vi "get_node_attribute.vi"(7 "attribute-name":string, 8 "error in (no error)":errorcluster, 9 "default value (empty variant)":variant, 10 "node":refnum<class "Node.lvclass">, 11 "graph":refnum<class "Graph.lvclass">) -> (0 "error out":errorcluster, 1 "attribute-value":variant, 2 "attribute found":bool, 3 "graph-out":refnum<class "Graph.lvclass">)   [LabVIEW 2020, in "graph.lvlib" / "Graph.lvclass"]
uses:
  Graph.lvclass
  Node/Node.lvclass
  Node/Node.lvclass/Node.ctl
  Graph.lvclass/Graph.ctl
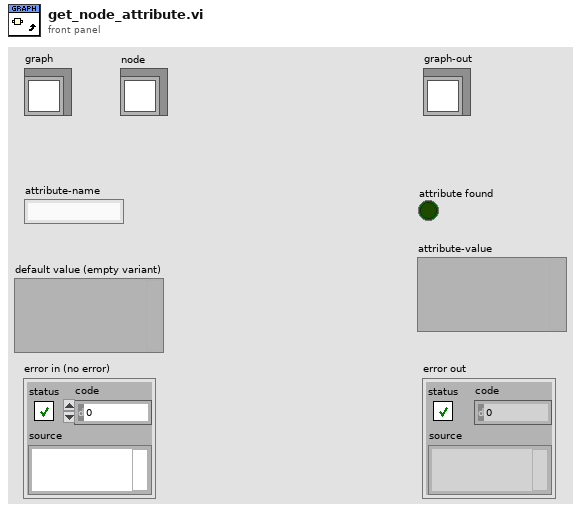
[diagram p1: front panel]
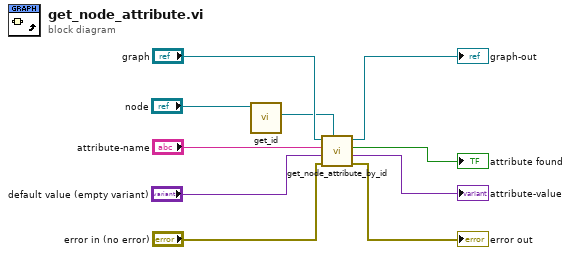
[diagram p0: block diagram]
diagram:
  n1 = call "get_id.vi"("node"="node") -> ("node-id"=w1:refnum<class "ID.lvclass">)  [unwired: 10 in]
  n2 = call "get_node_attribute_by_id.vi"("node-id"=w1, "error in (no error)"="error in (no error)", "default value (empty variant) in"="default value (empty variant)", "attribute-name"="attribute-name", "Graph in"="graph") -> ("error out"=→"error out":errorcluster, "default value (empty variant) out"=→"attribute-value":variant, "Boolean"=→"attribute found":bool, "Graph out"=→"graph-out":refnum<class "Graph.lvclass">)  [unwired: 3 in]
